vi "Main.vi"() -> ()   [LabVIEW 2014]
doc: "Showcases the API for manipulating the Windows task bar.\n\n\nCopyright (c) 2019 Sze Howe Koh.\nThis code is licensed under the MIT license."
uses:
  Command.ctl
  State.ctl
  <vilib>/addons/LQ/LQ Core/QSize.ctl
  <vilib>/addons/LQ/LQ Core/Qt/AlignmentFlag.ctl
  <vilib>/addons/LQ/Qt Widgets/QLabel/setWordWrap.vi
  <vilib>/addons/LQ/Qt Widgets/QWidget/setVisible.vi
  <vilib>/addons/LQ/Qt Widgets/QWidget/resize.vi
  <vilib>/addons/LQ/Qt Widgets/QLabel/setAlignment.vi
  <vilib>/addons/LQ/Qt Windows Extras/QWinTaskbarProgress/setValue.vi
  <vilib>/addons/LQ/Qt Windows Extras/QWinTaskbarProgress/setVisible.vi
  <vilib>/addons/LQ/Qt Windows Extras/QWinTaskbarProgress/value.vi
  <vilib>/addons/LQ/LQ Core/LQCoreEngine/_Polymorphic Instances/Connect_EventRefOut_Void.vi
  <vilib>/addons/LQ/LQ Core/LQCoreEngine/LQCoreEngine.lvclass
  <vilib>/addons/LQ/Qt Windows Extras/QWinThumbnailToolBar/QWinThumbnailToolBar.lvclass
  <vilib>/addons/LQ/Qt Windows Extras/QWinThumbnailToolButton/QWinThumbnailToolButton.lvclass
  <vilib>/addons/LQ/Qt GUI/QWindow/QWindow.lvclass
  <vilib>/addons/LQ/Qt Windows Extras/QWinTaskbarButton/QWinTaskbarButton.lvclass
  <vilib>/addons/LQ/Qt GUI/QIcon/QIcon.lvclass
  <vilib>/addons/LQ/Qt Widgets/QWidget/QWidget.lvclass
  <vilib>/addons/LQ/Qt Windows Extras/QWinTaskbarProgress/QWinTaskbarProgress.lvclass
  <vilib>/addons/LQ/Qt Widgets/QLabel/QLabel.lvclass
  <vilib>/addons/LQ/LQ Core/Qt/Qt.lvlib
panel:
  in  "Quit Button":bool
  # "Prerequisite knowledge/experience\n- \"Hello World - Multilingual Greetings (UTF-8)\", OR\n   Example 1. Constructing and Using a Widget from \"Hello World - Introduction to Widgets\"\n\n- LabVIEW Queued State Machine Architecture\n   https://decibel.ni.com/content/docs/DOC-32964\n\n\nInstructions\n1. Run this VI\n2. Hover your mouse cursor over the taskbar icon\n3. Click on the \"Play\", \"Pause\", \"Stop\", and \"Reset\" buttons in the taskbar\n\n\nShowcase\n- API for manipulating the Windows task bar\n\n\nKnown issues\n- After starting and stopping this VI (or any other VI that uses LQ), you must fully unload and\n   reload the DLLs first in order to run this example again (e.g. by restarting LabVIEW)"
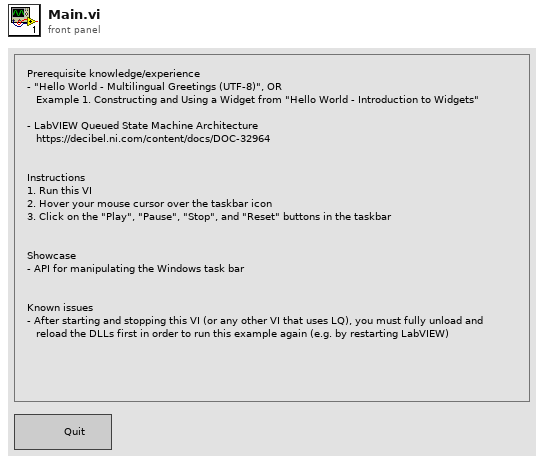
[diagram p1: front panel]
types:
  T1 = typedef "State.ctl" = enum16{"Idle", "Starting", "Active", "Pausing", "Paused", "Stopping", "Stopped", "Resetting"}
  T2 = typedef "Command.ctl" = enum16{"(Null)", "Play", "Pause", "Stop", "Reset"}
  T3 = typedef "QSize.ctl" = cluster{"width":i32, "height":i32}
  T4 = typedef "Qt.lvlib/AlignmentFlag.ctl" = i32
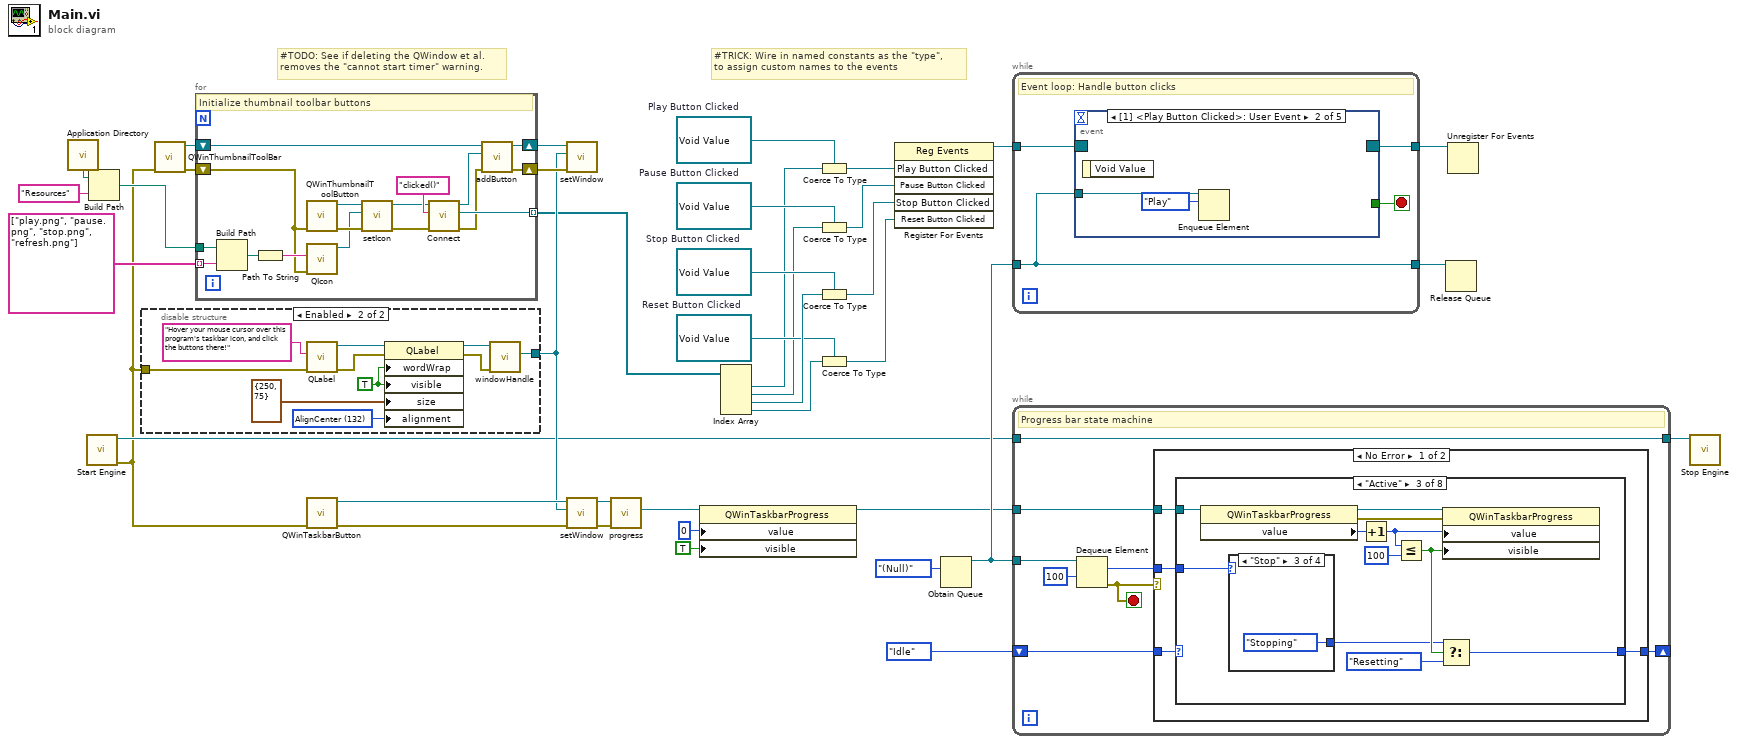
[diagram p0: block diagram]
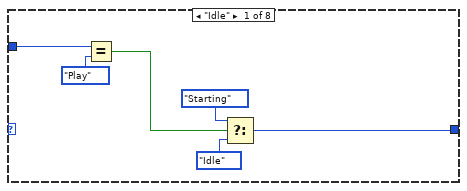
[diagram p2: hidden frame]
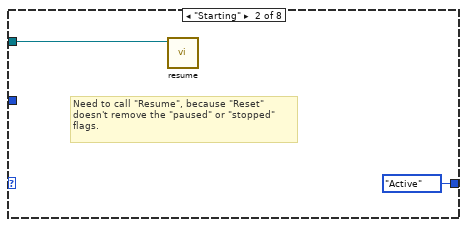
[diagram p3: hidden frame]
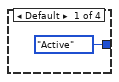
[diagram p4: hidden frame]
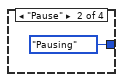
[diagram p5: hidden frame]
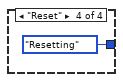
[diagram p6: hidden frame]
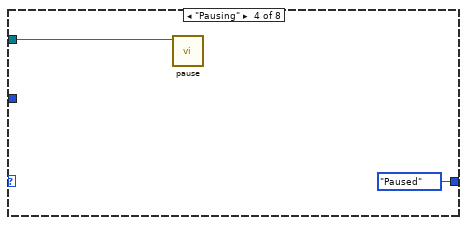
[diagram p7: hidden frame]
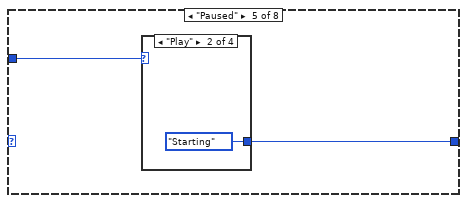
[diagram p8: hidden frame]
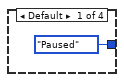
[diagram p9: hidden frame]
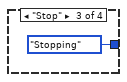
[diagram p10: hidden frame]
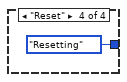
[diagram p11: hidden frame]
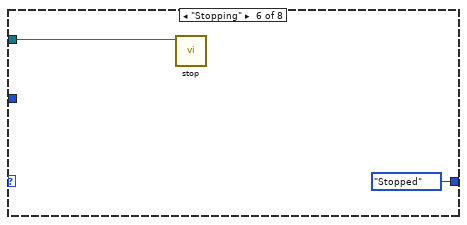
[diagram p12: hidden frame]
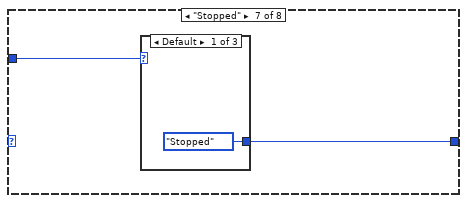
[diagram p13: hidden frame]
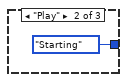
[diagram p14: hidden frame]
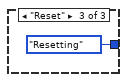
[diagram p15: hidden frame]
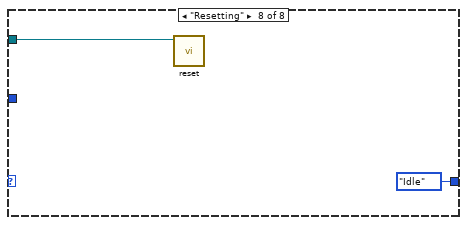
[diagram p16: hidden frame]
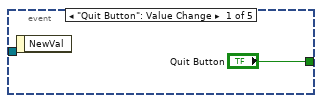
[diagram p18: hidden frame]
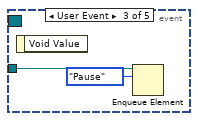
[diagram p19: hidden frame]
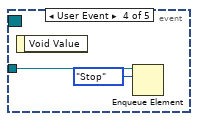
[diagram p20: hidden frame]
diagram:
  w9 = refnum<user-event> refnum  # Reset Button Clicked
  w12 = refnum<user-event> refnum  # Stop Button Clicked
  w7 = refnum<user-event> refnum  # Pause Button Clicked
  w8 = refnum<user-event> refnum  # Play Button Clicked
  # "#TRICK: Wire in named constants as the \"type\",\nto assign custom names to the events"
  # "#TODO: See if deleting the QWindow et al.\nremoves the \"cannot start timer\" warning."
  n1 = call <vilib>:"Application Directory.vi"() -> ("Application Directory"=w26:path)
  n2 = call <vilib>:"Start Engine.vi"() -> ("Error Out"=w13:errorcluster, "New Engine"=w19:refnum<class "LQCoreEngine.lvclass">)  [unwired: 10 in]
  n3 = Build Path(base path=w26, name or relative path="Resources") -> (appended path=w23:path)
  n4 = disable-structure shown="Enabled" {
    disable-tunnel: [w42 w54] -> w37
    disable-tunnel: w13 -> [w41 w49]
    frame Disabled {
      # "Thumbnail tool buttons currently can't be applied foreign\nwindows... :-/ (Bug in Qt?) Progress bar works fine though."
      n5 = control-ref of="This VI"() -> (w40:refnum<vi>)
      n6 = property class="VI"(reference=w40, error in=w41) -> (error out=w44:errorcluster, "FP.NativeWindow"=w43:u64)  [unwired: 1 out]
      n7 = call <vilib>:"fromWinId.vi"("Error In"=w44, "id"=w43) -> ("Value"=w42:refnum<class "QWindow.lvclass">)  [unwired: 8 in, 1 out]
    }
    frame Enabled {
      w46 = T4 132 items=["AlignLeft"=1, "AlignRight"=2, "AlignHCenter"=4, "AlignJustify"=8, "AlignAbsolute"=16, "AlignHorizontal_Mask"=31, "AlignTop"=32, "AlignBottom"=64, "AlignVCenter"=128, "AlignBaseline"=256, "AlignVertical_Mask"=480, "AlignCenter"=132] ("alignment")
      w45 = TRUE ("wordWrap")
      n8 = call <vilib>:"QLabel.vi"("Error In"=w49, "text"="Hover your mouse cursor over this program's taskbar icon, and click the buttons there!") -> ("Error Out"=w51:errorcluster, "New QLabel"=w53:refnum<class "QLabel.lvclass">)  [unwired: 8 in]
      n9 = property class="QLabel"(reference=w53, error in=w51, "wordWrap"=w45, "visible"=w45, "size"=T3 {"width"=250, "height"=75}, "alignment"=w46) -> (reference out=w52:refnum<class "QLabel.lvclass">, error out=w50:errorcluster)
      n10 = call <vilib>:"windowHandle.vi"("Error In"=w50, "QWidget In"=w52) -> ("Value"=w54:refnum<class "QWindow.lvclass">)  [unwired: 7 in, 2 out]
    }
  }
  n11 = call <vilib>:"QWinThumbnailToolBar.vi"("Error In"=w13) -> ("Error Out"=w24:errorcluster, "New QWinThumbnailToolBar"=w36:refnum<class "QWinThumbnailToolBar.lvclass">)  [unwired: 9 in]
  n12 = for {
    tunnel: [w66] -> w20 mode=indexing
    shift-right: [w69] -> w35
    shift-left: w36 -> [w70]
    tunnel: w23 -> [w61]
    tunnel: string[] ["play.png", "pause.png", "stop.png", "refresh.png"] -> [w60] mode=indexing
    shift-right: [w55] -> w39
    shift-left: w24 -> [w57]
    # "Initialize thumbnail toolbar buttons"
    n13 = Build Path(base path=w61, name or relative path=w60) -> (appended path=w59:path)
    n14 = Path To String(path=w59) -> (string=w58:string)
    n15 = call <vilib>:"QWinThumbnailToolButton.vi"("Error In"=w57) -> ("Error Out"=w71:errorcluster, "New QWinThumbnailToolButton"=w65:refnum<class "QWinThumbnailToolButton.lvclass">)  [unwired: 9 in]
    n16 = call <vilib>:"QIcon.vi"("Error In"=w57, "fileName"=w58) -> ("New QIcon"=w64:refnum<class "QIcon.lvclass">)  [unwired: 8 in, 1 out]
    n17 = call <vilib>:"setIcon.vi"("Error In"=w71, "icon"=w64, "QWinThumbnailToolButton In"=w65) -> ("Error Out"=w63:errorcluster, "QWinThumbnailToolButton Out"=w62:refnum<class "QWinThumbnailToolButton.lvclass">)  [unwired: 7 in]
    n18 = call-poly <vilib>:"Connect.vi"("Error In"=w63, "Signal Signature"="clicked()" ("Signal"), "Sender In"=w62) -> ("Error Out"=w56:errorcluster, "Void Signal"=w66:refnum<user-event>, "Sender Out"=w68:refnum<class "QWinThumbnailToolButton.lvclass">)  [unwired: 6 in]
    n19 = call <vilib>:"addButton.vi"("Error In"=w56, "button"=w68, "QWinThumbnailToolBar In"=w70) -> ("Error Out"=w55:errorcluster, "QWinThumbnailToolBar Out"=w69:refnum<class "QWinThumbnailToolBar.lvclass">)  [unwired: 7 in]
  }
  n20 = call <vilib>:"QWinTaskbarButton.vi"("Error In"=w13) -> ("Error Out"=w34:errorcluster, "New QWinTaskbarButton"=w38:refnum<class "QWinTaskbarButton.lvclass">)  [unwired: 9 in]
  n21 = call <vilib>:"setWindow.vi"("Error In"=w39, "window"=w37, "QWinThumbnailToolBar In"=w35) -> ()  [unwired: 7 in, 2 out]
  n22 = call <vilib>:"setWindow.vi"("Error In"=w34, "window"=w37, "QWinTaskbarButton In"=w38) -> ("Error Out"=w27:errorcluster, "QWinTaskbarButton Out"=w28:refnum<class "QWinTaskbarButton.lvclass">)  [unwired: 7 in]
  n23 = call <vilib>:"progress.vi"("Error In"=w27, "QWinTaskbarButton In"=w28) -> ("Value"=w15:refnum<class "QWinTaskbarProgress.lvclass">)  [unwired: 7 in, 2 out]
  n24 = property class="QWinTaskbarProgress"(reference=w15, "value"=0, "visible"=TRUE) -> (reference out=w14:refnum<class "QWinTaskbarProgress.lvclass">)  [unwired: 1 in, 1 out]
  n25 = Index Array(array=w20) -> (element #1=w4:refnum<user-event>, element #2=w5:refnum<user-event>, element #3=w11:refnum<user-event>, element #4=w6:refnum<user-event>)  [unwired: 4 in]
  n26 = Coerce To Type(0:w4, 1:w8) -> (2:w3:refnum<user-event>)
  n27 = Coerce To Type(0:w5, 1:w7) -> (2:w2:refnum<user-event>)
  n28 = Coerce To Type(0:w11, 1:w12) -> (2:w10:refnum<user-event>)
  n29 = Coerce To Type(0:w6, 1:w9) -> (2:w1:refnum<user-event>)
  n30 = register-events(w3, w2, w10, w1) -> (reference out=w33:refnum<event-registration>)  [unwired: 2 in, 1 out]
  n31 = Obtain Queue(element data type=Command."(Null)" ("Command")) -> (queue out=w21:refnum<queue>)  [unwired: 4 in, 2 out]
  n32 = while {
    tunnel: w33 -> [w75]
    tunnel: [w74] -> w32
    tunnel: [w72] -> w29
    tunnel: w21 -> [w72]
    stop <- w73 stop-if-true
    # "Event loop: Handle button clicks"
    n33 = event shown="[1] <Play Button Clicked>: User Event" {
      selector: w75 -> [_ _ _ _ _]
      dyn-events: [_ _ _ _ _] -> w74
      timeout: _ -> [_ _ _ _ _]
      tunnel: ["Quit Button" _ _ _ _] -> w73
      tunnel: w72 -> [_ w78 w80 w82 w84]
      event "Quit Button": Value Change {
        n34 = event-data() -> ()  [unwired: 1 in, 1 out]
      }
      event User Event {
        n35 = event-data() -> ()  [unwired: 1 in, 1 out]
        n36 = Enqueue Element(queue=w78, element=Command."Play") -> ()  [unwired: 2 in, 3 out]
      }
      event User Event {
        n37 = event-data() -> ()  [unwired: 1 in, 1 out]
        n38 = Enqueue Element(queue=w80, element=Command."Pause") -> ()  [unwired: 2 in, 3 out]
      }
      event User Event {
        n39 = event-data() -> ()  [unwired: 1 in, 1 out]
        n40 = Enqueue Element(queue=w82, element=Command."Stop") -> ()  [unwired: 2 in, 3 out]
      }
      event User Event {
        n41 = event-data() -> ()  [unwired: 1 in, 1 out]
        n42 = Enqueue Element(queue=w84, element=Command."Reset") -> ()  [unwired: 2 in, 3 out]
      }
    }
  }
  n43 = while {
    tunnel: w21 -> [w92]
    shift-right: [w87] -> _
    shift-left: State."Idle" ("State") -> [w88]
    tunnel: w14 -> [w86]
    tunnel: [w85] -> w18
    tunnel: w19 -> [w85]
    stop <- w90 stop-if-true
    # "Progress bar state machine"
    n44 = Dequeue Element(queue=w92, timeout in ms (-1)=100) -> (element=w89:T2, error out=w90:errorcluster)  [unwired: 1 in, 2 out]
    n45 = case shown="No Error" w90 {
      tunnel: w89 -> [w94 _]
      tunnel: w88 -> [w96 w137]
      tunnel: [w95 w137] -> w87
      tunnel: w86 -> [w93 _]
      frame No Error {
        n46 = case shown="\"Active\"" w96 {
          tunnel: [w98 State."Active" ("State") w107 State."Paused" ("State") w122 State."Stopped" ("State") w130 State."Idle" ("State")] -> w95
          tunnel: w94 -> [w102 _ w106 _ w123 _ w131 _]
          tunnel: w93 -> [_ w103 w115 w121 _ w129 _ w136]
          frame "Idle" {
            n47 = Equal?(x=w102, y=Command."Play") -> (x = y?=w97:bool)
            n48 = Select(t=State."Starting" ("State"), s=w97, f=State."Idle" ("State")) -> (s? t:f=w98:T1)
          }
          frame "Starting" {
            # "Need to call \"Resume\", because \"Reset\"\ndoesn't remove the \"paused\" or \"stopped\"\nflags."
            n49 = call <vilib>:"resume.vi"("QWinTaskbarProgress In"=w103) -> ()  [unwired: 9 in, 2 out]
          }
          frame "Active" {
            n50 = property class="QWinTaskbarProgress"(reference=w115) -> (reference out=w114:refnum<class "QWinTaskbarProgress.lvclass">, error out=w113:errorcluster, "value"=w112:i32)  [unwired: 1 in]
            n51 = case shown="\"Stop\"" w106 {
              tunnel: [State."Active" ("State") State."Pausing" ("State") State."Stopping" ("State") State."Resetting" ("State")] -> w105
              frame Default {
              }
              frame "Pause" {
              }
              frame "Stop" {
              }
              frame "Reset" {
              }
            }
            n52 = Increment(x=w112) -> (x+1=w111:i32)
            n53 = Less Or Equal?(x=w111, y=100) -> (x <= y?=w109:bool)
            n54 = Select(t=w105, s=w109, f=State."Resetting" ("State")) -> (s? t:f=w107:T1)
            n55 = property class="QWinTaskbarProgress"(reference=w114, error in=w113, "value"=w111, "visible"=w109) -> ()  [unwired: 2 out]
          }
          frame "Pausing" {
            n56 = call <vilib>:"pause.vi"("QWinTaskbarProgress In"=w121) -> ()  [unwired: 9 in, 2 out]
          }
          frame "Paused" {
            n57 = case shown="\"Play\"" w123 {
              tunnel: [State."Paused" ("State") State."Starting" ("State") State."Stopping" ("State") State."Resetting" ("State")] -> w122
              frame Default {
              }
              frame "Play" {
              }
              frame "Stop" {
              }
              frame "Reset" {
              }
            }
          }
          frame "Stopping" {
            n58 = call <vilib>:"stop.vi"("QWinTaskbarProgress In"=w129) -> ()  [unwired: 9 in, 2 out]
          }
          frame "Stopped" {
            n59 = case shown="Default" w131 {
              tunnel: [State."Stopped" ("State") State."Starting" ("State") State."Resetting" ("State")] -> w130
              frame Default {
              }
              frame "Play" {
              }
              frame "Reset" {
              }
            }
          }
          frame "Resetting" {
            n60 = call <vilib>:"reset.vi"("QWinTaskbarProgress In"=w136) -> ()  [unwired: 9 in, 2 out]
          }
        }
      }
      frame Error {
      }
    }
  }
  n61 = Release Queue(queue=w29) -> ()  [unwired: 2 in, 3 out]
  n62 = Unregister For Events(event registration refnum=w32) -> ()  [unwired: 1 in, 1 out]
  n63 = call <vilib>:"Stop Engine.vi"("LQCoreEngine"=w18) -> ()  [unwired: 10 in, 1 out]
